vi "Add Block Diagram Content.vi"(8 "error in (no error)":errorcluster, 9 "Term Refnum":refnum<vi>, 10 "ModuleLoop":T1, 11 "EST Digital Event in":refnum<class "Digital Event.lvclass">) -> (0 "error out":errorcluster, 3 "EST Digital Event out":refnum<class "Digital Event.lvclass">)   [LabVIEW 2015, in "Digital Event.lvclass"]
uses:
  Digital Event.lvclass
  VI/VI/Module.Refs.ctl
  <vilib>/Utility/miscctls.llb/LVPointTypeDef.ctl
  <vilib>/_script/New VI Object TypeDefs/NewVIObject_LVRelativePositionTypeDef.ctl
  <vilib>/_script/New VI Object TypeDefs/NewVIObject_LVRelativeDirectionTypeDef.ctl
  <vilib>/Utility/miscctls.llb/LVPoint32TypeDef.ctl
  Read Events.vi
  Signal/Read IP Core Path.vi
  Signal/Read Signal Name.vi
  Read Capture Path.vi
  VI/VI/VI.lvclass
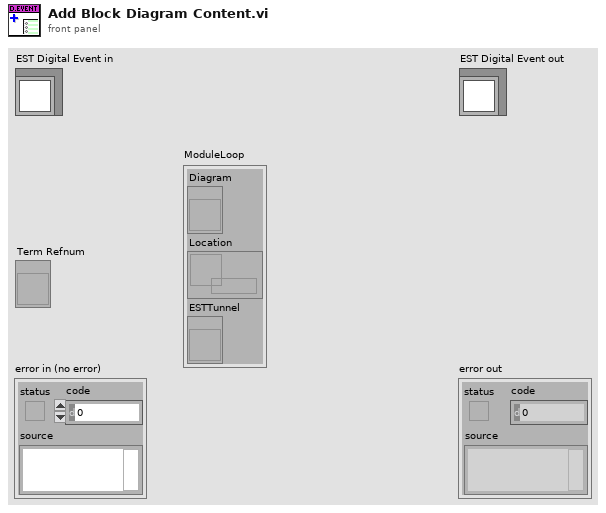
[diagram p1: front panel]
types:
  T1 = typedef "VI.lvclass/Module.Refs.ctl" = cluster{"Diagram":refnum<vi>, "Location":refnum<data-value>, "ESTTunnel":refnum<vi>}
  T2 = typedef "NewVIObject_LVRelativePositionTypeDef.ctl" = cluster{"Refnum":refnum<vi>, "Relative Direction":T3, "Point32":T4}
  T3 = typedef "NewVIObject_LVRelativeDirectionTypeDef.ctl" = enum32{"Right", "Left", "Top", "Bottom", "Top Right", "Top Left", "Bottom Right", "Bottom Left"}
  T4 = typedef "LVPoint32TypeDef.ctl" = cluster{"Horizontal":i32, "Vertical":i32}
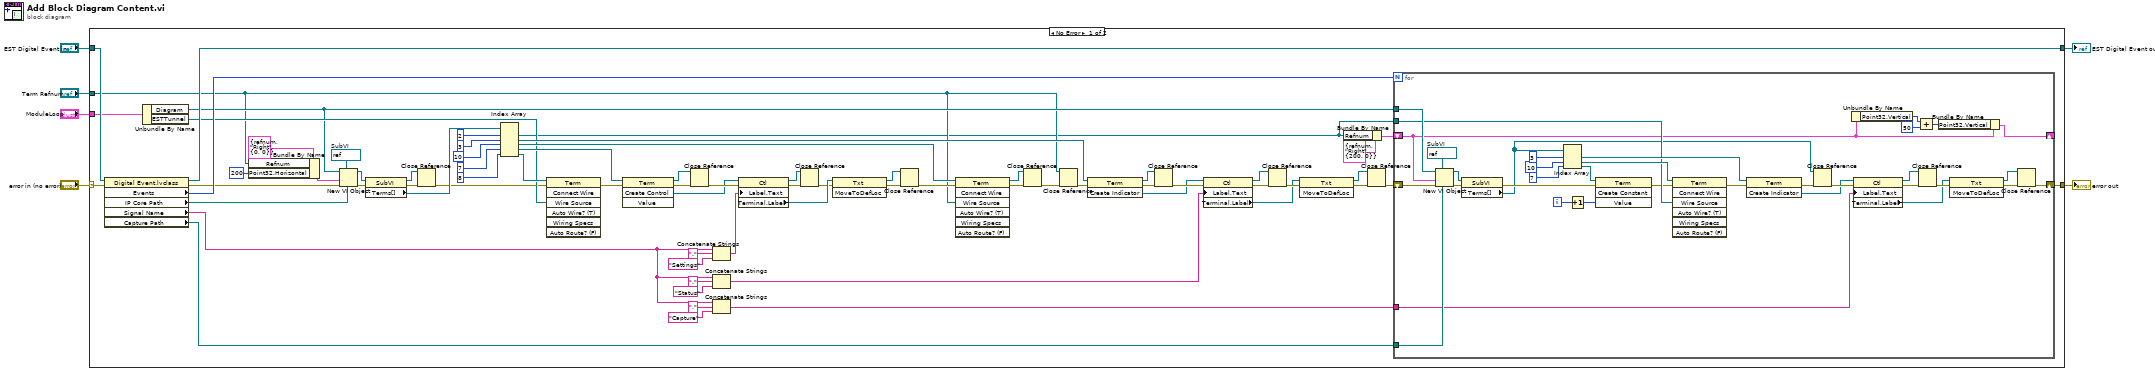
[diagram p0: block diagram]
diagram:
  n1 = case shown="No Error" "error in (no error)" {
    selector: "error in (no error)" -> [w10 w114]
    tunnel: "EST Digital Event in" -> [w29 w113]
    tunnel: [w25 w114] -> w5
    tunnel: [w24 w113] -> w4
    tunnel: "ModuleLoop" -> [w23 _]
    tunnel: "Term Refnum" -> [w19 _]
    frame No Error {
      w56 = refnum<vi> refnum  # SubVI
      n2 = property class="Digital Event.lvclass"(reference=w29, error in=w10) -> (reference out=w24:refnum<class "Digital Event.lvclass">, error out=w16:errorcluster, "Events"=w28:u32, "IP Core Path"=w11:path, "Signal Name"=w27:string, "Capture Path"=w26:path)
      n3 = Unbundle By Name(w23) -> ("Diagram"=w21:refnum<vi>, "ESTTunnel"=w22:refnum<vi>)
      n4 = Bundle By Name(cluster=T2 {"Refnum"=refnum, "Relative Direction"=enum."Right", "Point32"={"Horizontal"=0, "Vertical"=0}} ("Relative Position"), "Refnum"=w19, "Point32.Horizontal"=200) -> (w17:T2)
      n5 = New VI Object(vi object class=w56, owner refnum=w21, position/next to=w17, 6:w11, 8:w16) -> (object refnum=w58:refnum<vi>, 0:w59:errorcluster)  [unwired: 3 in]
      n6 = property class="SubVI"(reference=w58, error in=w59) -> (reference out=w9:refnum<vi>, error out=w8:errorcluster, "Terms[]"=w57:refnum<vi>[])
      n7 = Close Reference(reference=w9, error in (no error)=w8) -> (error out=w7:errorcluster)
      n8 = Index Array(array=w57, index #1=2 ("index"), index #2=3 ("index"), index #3=10 ("index"), index #4=7 ("index"), index #5=8 ("index")) -> (element #1=w14:refnum<vi>, element #2=w37:refnum<vi>, element #3=w38:refnum<vi>, element #4=w39:refnum<vi>, element #5=w31:refnum<vi>)
      n9 = invoke class="Term" method="Connect Wire"(reference=w31, error in=w7, "Wire Source"=w22) -> (error out=w30:errorcluster)  [unwired: 4 in, 6 out]
      n10 = invoke class="Term" method="Create Control"(reference=w39, error in=w30) -> (reference out=w67:refnum<vi>, error out=w66:errorcluster, "Create Control"=w55:refnum<vi>)  [unwired: 2 in, 1 out]
      n11 = Close Reference(reference=w67, error in (no error)=w66) -> (error out=w68:errorcluster)
      n12 = Concatenate Strings(w27, "." ("string"), "Settings" ("string")) -> (w60:string)
      n13 = Concatenate Strings(w27, "." ("string"), "Status" ("string")) -> (w36:string)
      n14 = Concatenate Strings(w27, "." ("string"), "Capture" ("string")) -> (w33:string)
      n15 = property class="Ctl"(reference=w55, error in=w68, "Label.Text"=w60) -> (reference out=w54:refnum<vi>, error out=w52:errorcluster, "Terminal.Label"=w53:refnum<vi>)
      n16 = Close Reference(reference=w54, error in (no error)=w52) -> (error out=w51:errorcluster)
      n17 = invoke class="Txt" method="MoveToDefLoc"(reference=w53, error in=w51) -> (reference out=w49:refnum<vi>, error out=w50:errorcluster)  [unwired: 1 in, 1 out]
      n18 = Close Reference(reference=w49, error in (no error)=w50) -> (error out=w48:errorcluster)
      n19 = invoke class="Term" method="Connect Wire"(reference=w38, error in=w48, "Wire Source"=w19) -> (reference out=w70:refnum<vi>, error out=w69:errorcluster)  [unwired: 4 in, 5 out]
      n20 = Close Reference(reference=w70, error in (no error)=w69) -> (error out=w71:errorcluster)
      n21 = Close Reference(reference=w19, error in (no error)=w71) -> (error out=w72:errorcluster)
      n22 = invoke class="Term" method="Create Indicator"(reference=w37, error in=w72) -> (reference out=w75:refnum<vi>, error out=w76:errorcluster, "Create Indicator"=w63:refnum<vi>)  [unwired: 1 in]
      n23 = Close Reference(reference=w75, error in (no error)=w76) -> (error out=w77:errorcluster)
      n24 = property class="Ctl"(reference=w63, error in=w77, "Label.Text"=w36) -> (reference out=w73:refnum<vi>, error out=w74:errorcluster, "Terminal.Label"=w45:refnum<vi>)
      n25 = Close Reference(reference=w73, error in (no error)=w74) -> (error out=w46:errorcluster)
      n26 = invoke class="Txt" method="MoveToDefLoc"(reference=w45, error in=w46) -> (reference out=w44:refnum<vi>, error out=w47:errorcluster)  [unwired: 1 in, 1 out]
      n27 = Bundle By Name(cluster=T2 {"Refnum"=refnum, "Relative Direction"=enum."Right", "Point32"={"Horizontal"=200, "Vertical"=0}} ("Relative Position"), "Refnum"=w14) -> (w13:T2)
      n28 = Close Reference(reference=w44, error in (no error)=w47) -> (error out=w12:errorcluster)
      n29 = for {
        N: w28 -> [_]
        shift-right: [w94] -> w25
        shift-left: w12 -> [w87]
        tunnel: w21 -> [w109]
        tunnel: w26 -> [w108]
        tunnel: w33 -> [w78]
        tunnel: w14 -> [w88]
        shift-right: [w82] -> _
        shift-left: w13 -> [w86]
        i -> [w91]
        w110 = refnum<vi> refnum  # SubVI
        n30 = New VI Object(vi object class=w110, owner refnum=w109, position/next to=w86, 6:w108, 8:w87) -> (object refnum=w111:refnum<vi>, 0:w112:errorcluster)  [unwired: 3 in]
        n31 = property class="SubVI"(reference=w111, error in=w112) -> (error out=w92:errorcluster, "Terms[]"=w79:refnum<vi>[])  [unwired: 1 out]
        n32 = Index Array(array=w79, index #1=3 ("index"), index #2=10 ("index"), index #3=7 ("index")) -> (element #1=w95:refnum<vi>, element #2=w89:refnum<vi>, element #3=w93:refnum<vi>)
        n33 = Increment(x=w91) -> (x+1=w90:i32)
        n34 = invoke class="Term" method="Create Constant"(reference=w93, error in=w92, "Value"=w90) -> (error out=w80:errorcluster)  [unwired: 1 in, 3 out]
        n35 = invoke class="Term" method="Connect Wire"(reference=w89, error in=w80, "Wire Source"=w88) -> (error out=w81:errorcluster)  [unwired: 4 in, 6 out]
        n36 = invoke class="Term" method="Create Indicator"(reference=w95, error in=w81) -> (error out=w103:errorcluster, "Create Indicator"=w100:refnum<vi>)  [unwired: 1 in, 1 out]
        n37 = Close Reference(reference=w79, error in (no error)=w103) -> (error out=w104:errorcluster)
        n38 = Unbundle By Name(w86) -> ("Point32.Vertical"=w85:i32)
        n39 = property class="Ctl"(reference=w100, error in=w104, "Label.Text"=w78) -> (reference out=w101:refnum<vi>, error out=w102:errorcluster, "Terminal.Label"=w97:refnum<vi>)
        n40 = Add(x=w85, y=50) -> (x+y=w83:i32)
        n41 = Close Reference(reference=w101, error in (no error)=w102) -> (error out=w98:errorcluster)
        n42 = Bundle By Name(cluster=w86, "Point32.Vertical"=w83) -> (w82:T2)
        n43 = invoke class="Txt" method="MoveToDefLoc"(reference=w97, error in=w98) -> (reference out=w96:refnum<vi>, error out=w99:errorcluster)  [unwired: 1 in, 1 out]
        n44 = Close Reference(reference=w96, error in (no error)=w99) -> (error out=w94:errorcluster)
      }
    }
    frame Error {
    }
  }
  "error out" <- w5
  "EST Digital Event out" <- w4
